vi "Generate IDs.vi"(4 "Type of Neuron":T1, 5 "Size":dbl) -> (0 "Possible IDs":i32[](array[numeric]))   [LabVIEW 2013]
doc: "Create the list of possible ids for neurons inside a given 3D grid"
uses:
  Controls/Type of Neuron.ctl
  <vilib>/Analysis/1siggen.llb/Riffle Array (I32).vi
  <vilib>/Analysis/NI_AALBase.lvlib
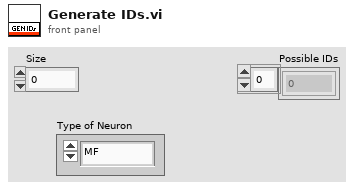
[diagram p1: front panel]
types:
  T1 = typedef "Type of Neuron.ctl" = enum16{"MF", "BA", "GO", "GC", "PC", "LU", "Glia (Dummy)"}
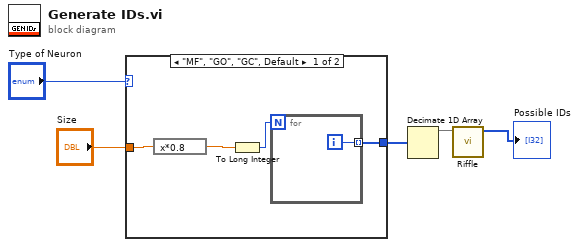
[diagram p0: block diagram]
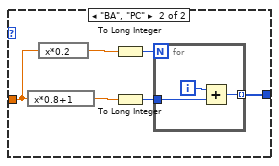
[diagram p2: hidden frame]
diagram:
  n1 = case shown="\"MF\", \"GO\", \"GC\", Default" "Type of Neuron" {
    tunnel: "Size" -> [w9 w14]
    tunnel: [w6 w11] -> w2
    frame "MF", "GO", "GC", Default {
      n2 = expression code="x*0.8"(w9) -> (w8:dbl)
      n3 = To Long Integer(number=w8) -> (32bit integer=w7:i32)
      n4 = for {
        N: w7 -> [_]
        tunnel: [w10] -> w6 mode=indexing
        i -> [w10]
      }
    }
    frame "BA", "PC" {
      n5 = expression code="x*0.8+1"(w14) -> (w16:dbl)
      n6 = expression code="x*0.2"(w14) -> (w13:dbl)
      n7 = To Long Integer(number=w13) -> (32bit integer=w12:i32)
      n8 = To Long Integer(number=w16) -> (32bit integer=w15:i32)
      n9 = for {
        N: w12 -> [_]
        tunnel: [w18] -> w11 mode=indexing
        tunnel: w15 -> [w17]
        i -> [w19]
        n10 = Add(x=w19, y=w17) -> (x+y=w18:i32)
      }
    }
  }
  n11 = Decimate 1D Array(w2) -> (w3:i32[])  [unwired: 3 out]
  n12 = call-poly <vilib>:"Riffle.vi"("X"=w3) -> ("Riffled {X}"=→"Possible IDs":i32[])  [unwired: 8 in, 2 out]
